vi "createTopicClusterControlRef.vi"(8 "error in (no error)":errorcluster, 11 "PolymorphicInstance in":refnum<class "PolymorphicInstance.lvclass">) -> (0 "error out":errorcluster, 3 "PolymorphicInstance out":refnum<class "PolymorphicInstance.lvclass">)   [LabVIEW 2013, in "PolymorphicInstance.lvclass"]
uses:
  PolymorphicInstance.lvclass
  PolymorphicInstance.lvclass/PolymorphicInstance.ctl
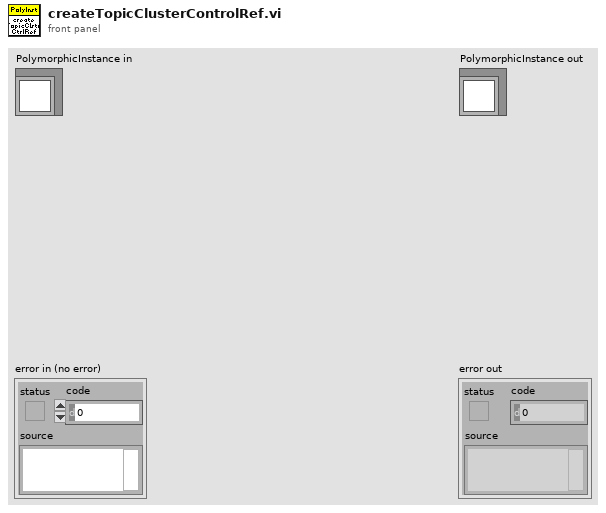
[diagram p1: front panel]
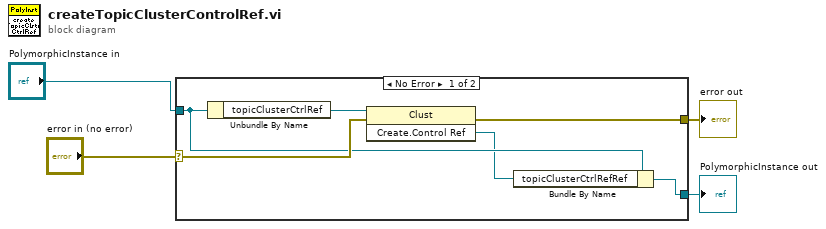
[diagram p0: block diagram]
diagram:
  n1 = case shown="No Error" "error in (no error)" {
    selector: "error in (no error)" -> [w9 w12]
    tunnel: [w8 w12] -> w3
    tunnel: [w6 w11] -> w1
    tunnel: "PolymorphicInstance in" -> [w7 w11]
    frame No Error {
      n2 = Unbundle By Name(w7) -> ("topicClusterCtrlRef"=w10:refnum<vi>)
      n3 = invoke class="Clust" method="Create.Control Ref"(reference=w10, error in=w9) -> (error out=w8:errorcluster, "Create Control Ref"=w5:refnum<vi>)  [unwired: 1 in, 1 out]
      n4 = Bundle By Name(cluster=w7, "topicClusterCtrlRefRef"=w5) -> (w6:refnum<class "PolymorphicInstance.lvclass">)
    }
    frame Error {
    }
  }
  "error out" <- w3
  "PolymorphicInstance out" <- w1
